vi "Start GNU Octave.vi"(7 "hide window (T)":bool=TRUE, 8 "error in":errorcluster, 10 "Octave binary directory":path, 11 "Working directory":path) -> (0 "error out":errorcluster, 1 "initial output":string, 2 "GNU Octave version":string, 3 "pipe out":T1)   [LabVIEW 2013, in "GOLPI library.lvlib"]
uses:
  GOLPI library.lvlib
  LV Process.lvlibp/Pipe Handle.ctl
  <vilib>/Utility/error.llb/Error Cluster From Error Code.vi
  <vilib>/ErrorRing/Error Ring.xnode
  <vilib>/regexp/Match Regular Expression.xnode
  LV Process.lvlibp
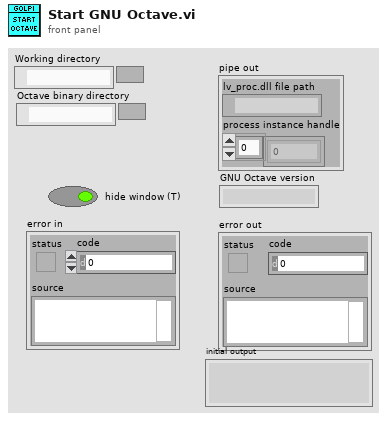
[diagram p1: front panel]
types:
  T1 = typedef "LV Process.lvlibp/Pipe Handle.ctl" = cluster{"lv_proc.dll file path":path, "process instance handle":u32[]}
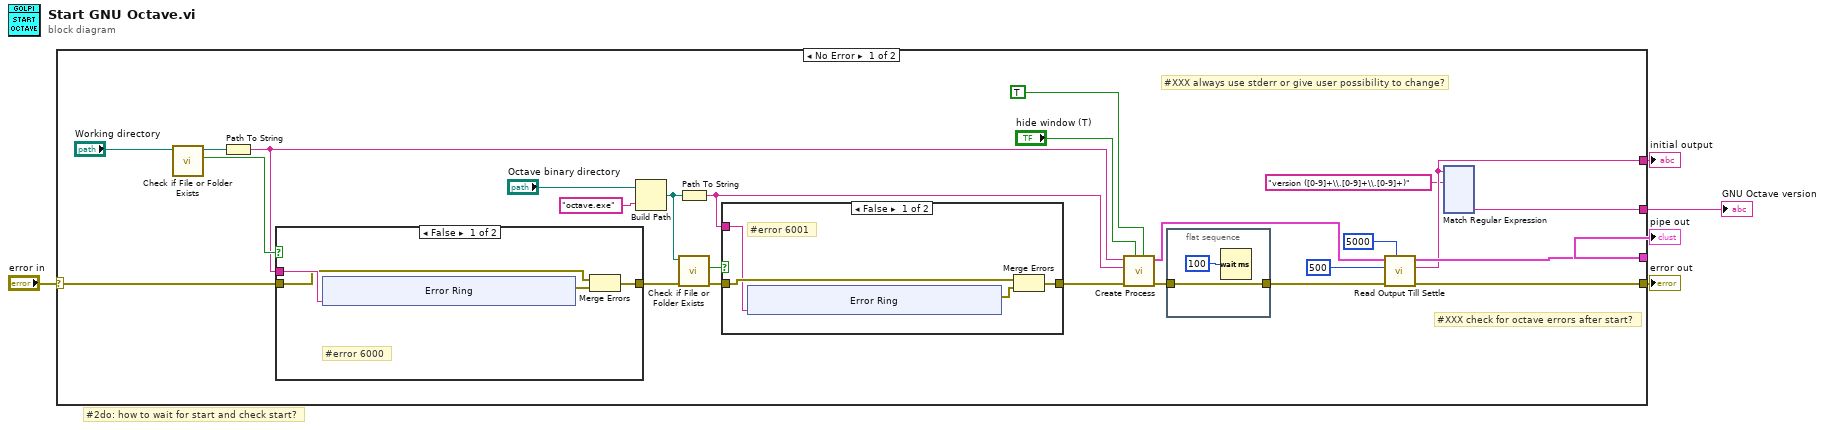
[diagram p0: block diagram]
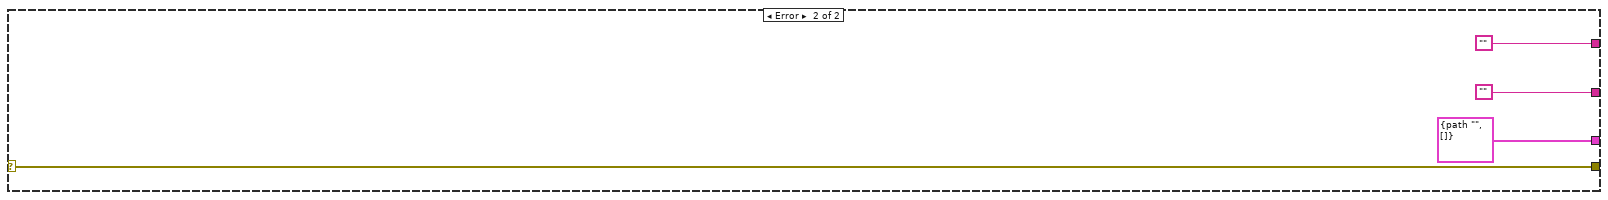
[diagram p4: hidden frame]
diagram:
  # "#2do: how to wait for start and check start?"
  n1 = case shown="No Error" "error in" {
    selector: "error in" -> [w20 w176]
    tunnel: [w10 w176] -> w4
    tunnel: [w9 T1 {"lv_proc.dll file path"=path "", "process instance handle"=[]} ("pipe handle")] -> w3
    tunnel: [w6 ""] -> w2
    tunnel: [w8 ""] -> w1
    frame No Error {
      # "#XXX check for octave errors after start?"
      # "#XXX always use stderr or give user possibility to change?"
      n2 = call <vilib>:"Check if File or Folder Exists.vi"("path"="Working directory") -> ("file or folder exists?"=w26:bool, "dup path"=w27:path)  [unwired: 8 in, 1 out]
      n3 = Path To String(path=w27) -> (string=w25:string)
      n4 = case shown="False" w26 {
        tunnel: [w161 w172] -> w24
        tunnel: w20 -> [w163 w172]
        tunnel: w25 -> [w164 _]
        frame False {
          # "#error 6000"
          n5 = xnode "Error Ring"("parameter 0"=w164) -> ("error out"=w162:errorcluster)
          n6 = Merge Errors(w163, w162) -> (w161:errorcluster)
        }
        frame True {
        }
      }
      n7 = Build Path(base path="Octave binary directory", name or relative path="octave.exe" ("string")) -> (appended path=w17:path)
      n8 = Path To String(path=w17) -> (string=w16:string)
      n9 = call <vilib>:"Check if File or Folder Exists.vi"("error in (no error)"=w24, "path"=w17) -> ("error out"=w22:errorcluster, "file or folder exists?"=w23:bool)  [unwired: 7 in, 1 out]
      n10 = case shown="False" w23 {
        tunnel: w22 -> [w151 w160]
        tunnel: [w150 w160] -> w21
        tunnel: w16 -> [w149 _]
        frame False {
          # "#error 6001"
          n11 = xnode "Error Ring"("parameter 0"=w149) -> ("error out"=w152:errorcluster)
          n12 = Merge Errors(w151, w152) -> (w150:errorcluster)
        }
        frame True {
        }
      }
      n13 = call "Create Process.vi"("use stderr (F)"=TRUE, "hide window (T)"="hide window (T)", "error in"=w21, "command"=w16, "working folder"=w25) -> ("error out"=w14:errorcluster, "pipe handle"=w15:T1)  [unwired: 5 in]
      n14 = flat-sequence {
        tunnel: [w147] -> w13
        tunnel: w14 -> [w147]
        frame #0 {
          n15 = Wait (ms)(milliseconds to wait=u32 100) -> ()  [unwired: 1 out]
        }
      }
      n16 = call "Read Output Till Settle.vi"("timeout [ms]"=u32 5000, "error in"=w13, "settled for [ms]"=u32 500, "pipe in"=w15) -> ("error out"=w10:errorcluster, "read buffer"=w8:string, "pipe out"=w9:T1)  [unwired: 4 in, 1 out]
      n17 = xnode "Match Regular Expression"("input string"=w8, "regular expression"="version ([0-9]+\\.[0-9]+\\.[0-9]+)") -> ("submatch 1"=w6:string)  [unwired: 4 in, 5 out]
    }
    frame Error {
    }
  }
  "error out" <- w4
  "pipe out" <- w3
  "GNU Octave version" <- w2
  "initial output" <- w1
